vi "Read 3D Bar Property Array.vi"(8 "error in (no error)":errorcluster, 11 "3D Bar.lvclass in":refnum<class "3D Bar.lvclass">) -> (0 "error out":errorcluster, 2 "3D Bar Property Array":T1, 3 "3D Bar.lvclass out":refnum<class "3D Bar.lvclass">)   [LabVIEW 2020, in "3D Bar.lvclass"]
uses:
  <vilib>/Math Plots/3D Math Plots/3D Bar/3D Bar/3D Bar.lvclass
  <vilib>/Math Plots/3D Math Plots/3D Bar/3D Bar/Typedef/3D Bar Property Array.ctl
  <vilib>/Math Plots/3D Math Plots/3D Bar/3D Bar/Typedef/3D Bar Property.ctl
  <vilib>/Math Plots/3D Math Plots/3D Plot/3D Plot/Typedef/Line Type.ctl
  <vilib>/Math Plots/3D Math Plots/3D Bar/3D Bar/3D Bar.lvclass/3D Bar.ctl
  <vilib>/Math Plots/3D Math Plots/3D Plot/3D Plot/3D Plot.lvclass
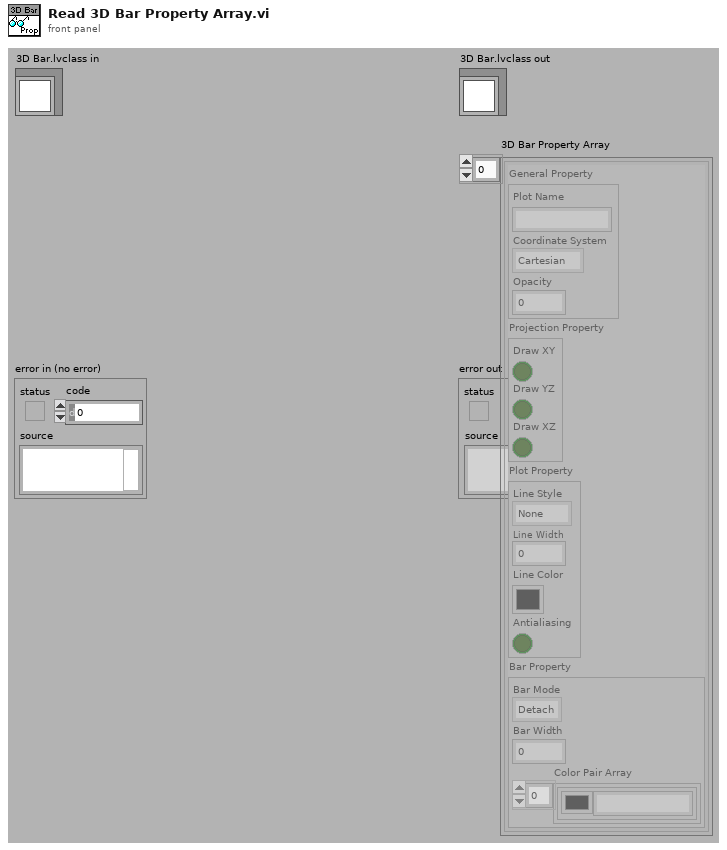
[diagram p1: front panel]
types:
  T1 = typedef "3D Bar.lvclass/3D Bar Property Array.ctl" = T2[]
  T2 = typedef "3D Bar.lvclass/3D Bar Property.ctl" = cluster{"General Property":cluster{"Plot Name":string, "Coordinate System":enum16{"Cartesian", "Cylindrical", "Spherical"}, "Opacity":sgl}, "Projection Property":cluster{"Draw XY":bool, "Draw YZ":bool, "Draw XZ":bool}, "Plot Property":cluster{"Line Style":T3, "Line Width":sgl, "Line Color":u32, "Antialiasing":bool}, "Bar Property":cluster{"Bar Mode":enum16{"Detach", "Group", "Stack"}, "Bar Width":sgl, "Color Pair Array":cluster{"Color":u32, "String":string}[]}}
  T3 = typedef "3D Plot.lvclass/Line Type.ctl" = enum16{"None", "Solid", "Dash", "Dot", "Dash Dot"}
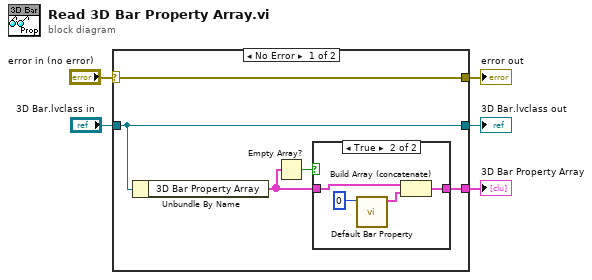
[diagram p0: block diagram]
diagram:
  n1 = case shown="No Error" "error in (no error)" {
    selector: "error in (no error)" -> [w10 w16]
    tunnel: [w10 w16] -> w4
    tunnel: [w9 w17] -> w2
    tunnel: "3D Bar.lvclass in" -> [w9 w17]
    tunnel: [w7 _] -> w1
    frame No Error {
      n2 = Unbundle By Name(w9) -> ("3D Bar Property Array"=w6:T1)
      n3 = Empty Array?(array=w6) -> (empty?=w8:bool)
      n4 = case shown="True" w8 {
        tunnel: [w11 w13] -> w7
        tunnel: w6 -> [w11 w15]
        frame False {
        }
        frame True {
          n5 = call <vilib>:"Default Bar Property.vi"("Plot ID"=0) -> ("Default Property"=w14:T2)  [unwired: 10 in]
          n6 = Build Array (concatenate)(w15, w14) -> (w13:T1)
        }
      }
    }
    frame Error {
    }
  }
  "error out" <- w4
  "3D Bar.lvclass out" <- w2
  "3D Bar Property Array" <- w1
